vi "Get Active Line UID.vi"(8 "error in (no error)":errorcluster, 11 "Pairing Tab Refs":T1) -> (0 "error out":errorcluster, 2 "Line UID":string)   [LabVIEW 2015, in "E2E Tag Exchange editor node.lvclass"]
uses:
  E2E Tag Exchange editor node.lvclass
  Pairing Tab References.ctl
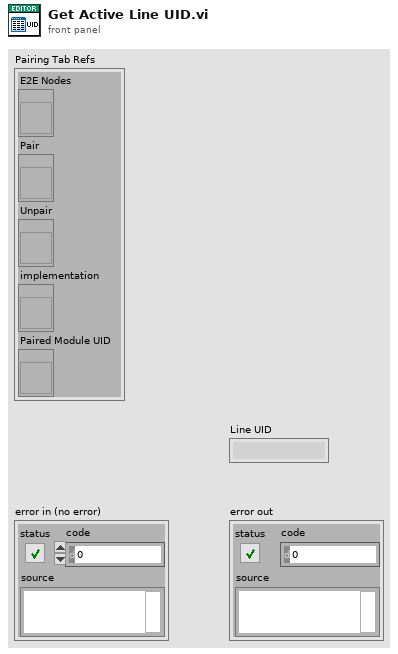
[diagram p1: front panel]
types:
  T1 = typedef "E2E Tag Exchange editor node.lvclass/Pairing Tab References.ctl" = cluster{"E2E Nodes":refnum<vi>, "Pair":refnum<vi>, "Unpair":refnum<vi>, "implementation":refnum<vi>, "Paired Module UID":refnum<vi>}
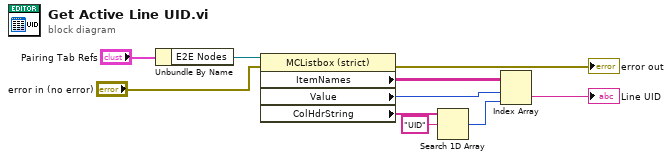
[diagram p0: block diagram]
diagram:
  n1 = Unbundle By Name("Pairing Tab Refs") -> ("E2E Nodes"=w9:refnum<vi>)
  n2 = property class="MCListbox (strict)"(reference=w9, error in="error in (no error)") -> (error out=→"error out":errorcluster, "ItemNames"=w6:string[][], "Value"=w5:i32, "ColHdrString"=w8:string[])  [unwired: 1 out]
  n3 = Search 1D Array(1D array=w8, element="UID") -> (index of element=w4:i32)  [unwired: 1 in]
  n4 = Index Array(array=w6, index (row)=w5, index (col)=w4) -> (element=→"Line UID":string)
